vi "LoadOneImageviaPath.vi"(1 "ImagePath":string="data path", 2 "ImageName":string=".jpg", 3 "error in (no error)":errorcluster) -> (8 "Image Out":T1, 9 "Image Pixels (U8)":u8[][](array[numeric]), 10 "error out":errorcluster)   [LabVIEW 2011, in "OfflineTracker.lvlib"]
uses:
  <vilib>/vision/Image Controls.llb/IMAQ Image.ctl
  OfflineTracker.lvlib
panel:
  out "image array out2":u8[][](graph)
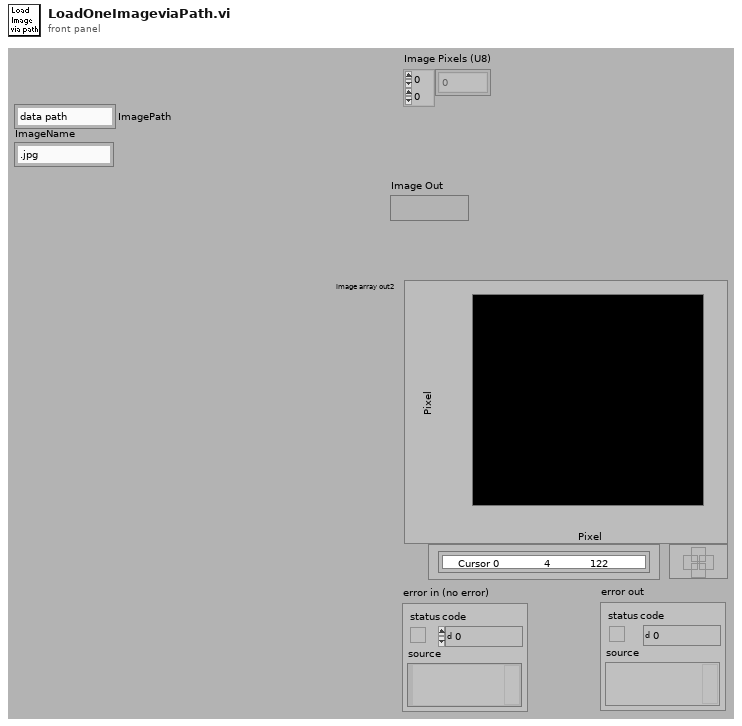
[diagram p1: front panel]
types:
  T1 = typedef "IMAQ Image.ctl" = refnum<image>
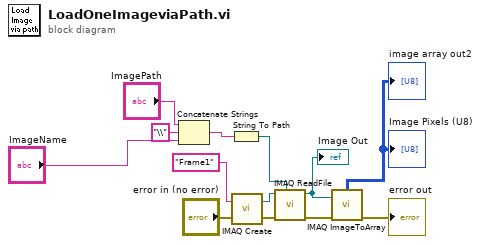
[diagram p0: block diagram]
diagram:
  n1 = Concatenate Strings("ImagePath", "\\" ("string"), "ImageName") -> (w7:string)
  n2 = String To Path(string=w7) -> (path=w8:path)
  n3 = call "IMAQ Create"("Image Name"="Frame1", "error in (no error)"="error in (no error)") -> ("New Image"=w10:T1, "error out"=w11:errorcluster)  [unwired: 2 in, 1 out]
  n4 = call "IMAQ ReadFile"("File Path"=w8, "error in (no error)"=w11, "Image"=w10) -> ("error out"=w12:errorcluster, "Image Out"=w13:T1)  [unwired: 2 in, 5 out]
  "Image Out" <- w13
  n5 = call "IMAQ ImageToArray"("error in (no error)"=w12, "Image"=w13) -> ("error out"=→"error out":errorcluster, "Image Pixels (U8)"=→"image array out2" →"Image Pixels (U8)":u8[][])  [unwired: 1 in, 4 out]
